vi "Restrict X Range (multiple).vi"(8 "error in (no error)":errorcluster, 9 "X Max":dbl, 10 "X Min":dbl, 11 "XY-data":cluster{"X-array":dbl[], "Y-array":dbl[]}[](array[cluster])) -> (0 "error out":errorcluster, 3 "XY-data out":cluster{"X-array":dbl[], "Y-array":dbl[]}[](array[cluster]) {"Y-array" format="%.2p"; "X-array" format="%.2p"})   [LabVIEW 2019, in "xy_utilities.lvlib"]
doc: "Removes data points that fall outside of the range defined by <b>x min</b> and <b>x max</b>\n\nWire data to the data input to determine the polymorphic instance to use or manually select the instance."
uses:
  xy_utilities.lvlib
  <vilib>/Analysis/6fits.llb/Remove Outliers.vi
  <vilib>/Analysis/6fits.llb/Remove Outliers (Range).vi
  <vilib>/Utility/error.llb/Error Cluster From Error Code.vi
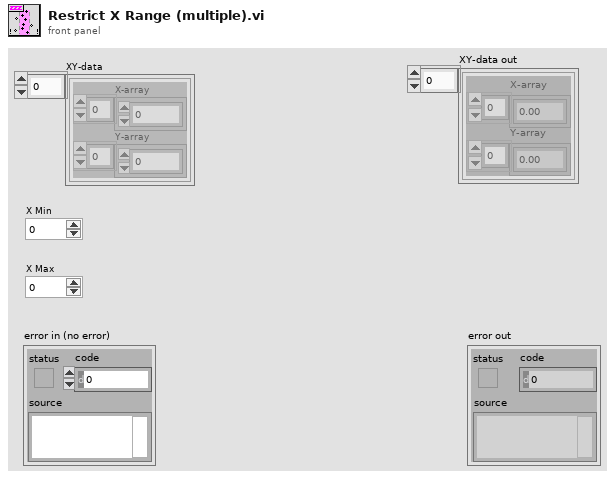
[diagram p1: front panel]
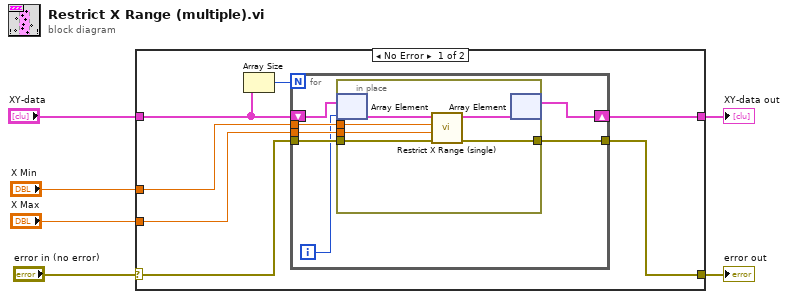
[diagram p0: block diagram]
diagram:
  n1 = case shown="No Error" "error in (no error)" {
    selector: "error in (no error)" -> [w12 w28]
    tunnel: [w11 w28] -> w5
    tunnel: "XY-data" -> [w7 w27]
    tunnel: [w13 w27] -> w3
    tunnel: "X Max" -> [w9 _]
    tunnel: "X Min" -> [w10 _]
    frame No Error {
      n2 = Array Size(array=w7) -> (size(s)=w8:i32)
      n3 = for {
        N: w8 -> [_]
        tunnel: w12 -> [w20]
        tunnel: [w19] -> w11
        tunnel: w10 -> [w18]
        tunnel: w9 -> [w17]
        shift-right: [w14] -> w13
        shift-left: w7 -> [w16]
        i -> [w15]
        n4 = in-place {
          in-place-border: w20 -> [w26]
          in-place-border: [w25] -> w19
          in-place-border: w18 -> [w24]
          in-place-border: w17 -> [w23]
          n5 = in-place-array #1(w16, w15) -> (w22:cluster{"X-array":dbl[], "Y-array":dbl[]})
          n6 = call "Restrict X Range (single).vi"("error in (no error)"=w26, "X Max"=w23, "X Min"=w24, "XY-data"=w22) -> ("error out"=w25:errorcluster, "XY-data out"=w21:cluster{"X-array":dbl[], "Y-array":dbl[]})  [unwired: 6 in]
          n7 = in-place-array #1(w21) -> (w14:cluster{"X-array":dbl[], "Y-array":dbl[]}[])  [unwired: 1 out]
        }
      }
    }
    frame Error {
    }
  }
  "error out" <- w5
  "XY-data out" <- w3
